vi "Get Process Model.vi"(8 "error in (no error)":errorcluster, 11 "SequenceFile in":refnum<class "SequenceFile.lvclass">) -> (0 "error out":errorcluster, 2 "Process Model":T1, 3 "SequenceFile out":refnum<class "SequenceFile.lvclass">)   [LabVIEW 2020, in "TSS.lvlib" / "SequenceFile.lvclass"]
uses:
  SequenceFile.lvclass
  Typedefs/Session Handle.ctl
  SequenceFile.lvclass/SequenceFile.ctl
  <vilib>/Utility/error.llb/Error Cluster From Error Code.vi
  <vilib>/ErrorRing/Error Ring.xnode
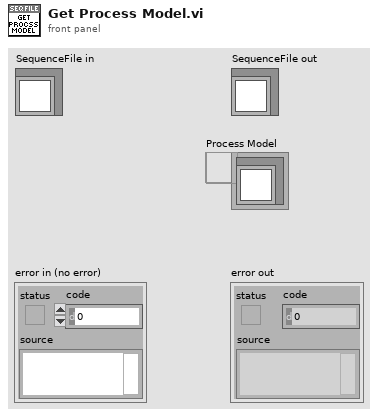
[diagram p1: front panel]
types:
  T1 = typedef "TSS.lvlib/SequenceFile.lvclass/Session Handle.ctl" = refnum<data-value>
  T2 = typedef "TSS.lvlib/Sequence File Type.ctl" = enum16{"Normal", "Model", "Front End Callbacks", "Station Callbacks", "Template"}
  T3 = typedef "TSS.lvlib/Engine.lvclass/Session Handle.ctl" = refnum<data-value>
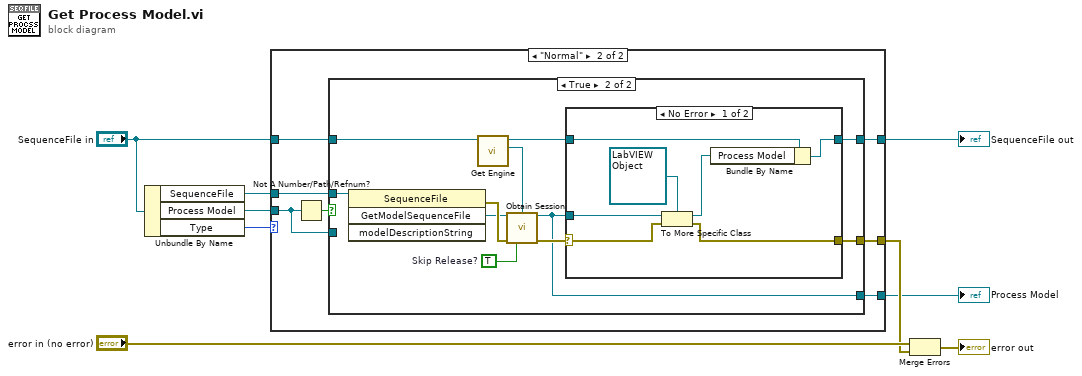
[diagram p0: block diagram]
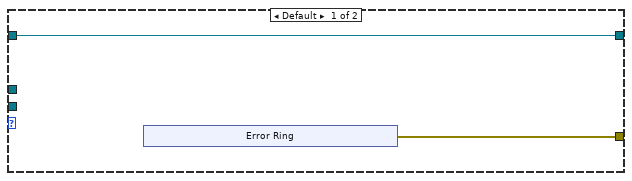
[diagram p2: hidden frame]
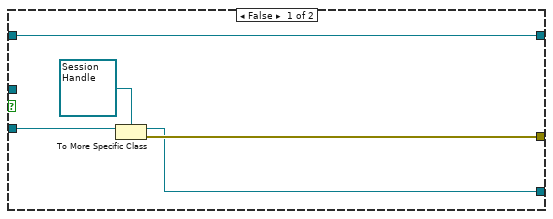
[diagram p3: hidden frame]
diagram:
  n1 = Unbundle By Name("SequenceFile in") -> ("SequenceFile"=w8:refnum<k7>, "Process Model"=w7:refnum<data-value>, "Type"=w2:T2)
  n2 = case shown="\"Normal\"" w2 {
    tunnel: w8 -> [_ w22]
    tunnel: w7 -> [_ w20]
    tunnel: [_ w19] -> w1
    tunnel: [w11 w18] -> w5
    tunnel: "SequenceFile in" -> [w10 w17]
    tunnel: [w10 w16] -> w3
    frame Default {
      n3 = xnode "Error Ring"() -> ("error out"=w11:errorcluster)
    }
    frame "Normal" {
      n4 = Not A Number/Path/Refnum?(number/path/refnum=w20) -> (NaN/Path/Refnum?=w21:bool)
      n5 = case shown="True" w21 {
        tunnel: w22 -> [_ w37]
        tunnel: w20 -> [w27 _]
        tunnel: [w23 w32] -> w19
        tunnel: [w25 w33] -> w18
        tunnel: w17 -> [w24 w31]
        tunnel: [w24 w35] -> w16
        frame False {
          n6 = To More Specific Class(target class=T1 refnum ("SequenceFile"), reference=w27) -> (specific class reference=w23:T1, error out=w25:errorcluster)  [unwired: 1 in]
        }
        frame True {
          w28 = TRUE  # Skip Release?
          n7 = invoke class="SequenceFile" method="GetModelSequenceFile"(reference=w37) -> (error out=w38:errorcluster, "GetModelSequenceFile"=w36:refnum<k7>)  [unwired: 3 in, 2 out]
          n8 = call "Get Engine.vi"("SequenceFile in"=w31) -> ("Engine"=w29:T3, "SequenceFile out"=w30:refnum<class "SequenceFile.lvclass">)  [unwired: 8 in, 1 out]
          n9 = call "Obtain Session.vi"("SequenceFile"=w36, "Engine"=w29, "error in (no error)"=w38, "Skip Release? (F)"=w28) -> ("Session Handle"=w32:T1, "error out"=w34:errorcluster)  [unwired: 10 in]
          n10 = case shown="No Error" w34 {
            selector: w34 -> [w40 w47]
            tunnel: w30 -> [w45 w46]
            tunnel: w32 -> [w44 _]
            tunnel: [w43 w46] -> w35
            tunnel: [w39 w47] -> w33
            frame No Error {
              n11 = To More Specific Class(target class=refnum<data-value> refnum, reference=w44, error in=w40) -> (specific class reference=w42:refnum<data-value>, error out=w39:errorcluster)
              n12 = Bundle By Name(cluster=w45, "Process Model"=w42) -> (w43:refnum<class "SequenceFile.lvclass">)
            }
            frame Error {
            }
          }
        }
      }
    }
  }
  "SequenceFile out" <- w3
  "Process Model" <- w1
  n13 = Merge Errors("error in (no error)", w5) -> (→"error out":errorcluster)
